vi "Delete all RT FIFOS.vi"(8 "error in":errorcluster, 11 "RT FIFOs--cluster":T1) -> (0 "error out":errorcluster)   [LabVIEW 2021, in "RT Main.lvlib"]
uses:
  RT Main.lvlib
  RT FIFOS--cluster.ctl
  Libraries/Common RT/Hardware Monitoring.ctl
  Libraries/Common RT/Common RT.lvlib
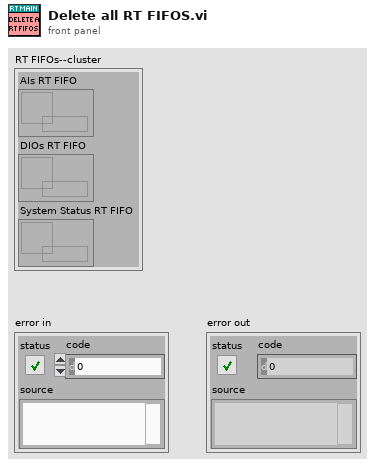
[diagram p1: front panel]
types:
  T1 = typedef "RT Main.lvlib/RT FIFOS--cluster.ctl" = cluster{"AIs RT FIFO":refnum<k33>, "DIOs RT FIFO":refnum<k33>, "System Status RT FIFO":refnum<k33>}
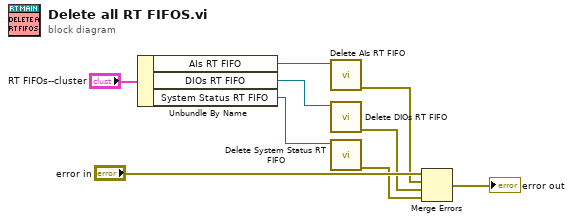
[diagram p0: block diagram]
diagram:
  n1 = Unbundle By Name("RT FIFOs--cluster") -> ("AIs RT FIFO"=w7:refnum<k33>, "DIOs RT FIFO"=w6:refnum<k33>, "System Status RT FIFO"=w5:refnum<k33>)
  n2 = call "Delete AIs RT FIFO.vi"("AIs RT FIFO"=w7) -> ("error out"=w1:errorcluster)  [unwired: 10 in]
  n3 = call "Delete DIOs RT FIFO.vi"("DIOs RT FIFO"=w6) -> ("error out"=w2:errorcluster)  [unwired: 10 in]
  n4 = call "Delete System Status RT FIFO.vi"("System Status RT FIFO"=w5) -> ("error out"=w3:errorcluster)  [unwired: 10 in]
  n5 = Merge Errors("error in", w1, w2, w3) -> (→"error out":errorcluster)
